vi "8.vi"() -> ()   [LabVIEW 2017]
panel:
  out "毫秒计时值":u32
  in  "开始":bool
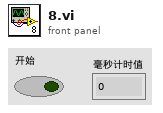
[diagram p1: front panel]
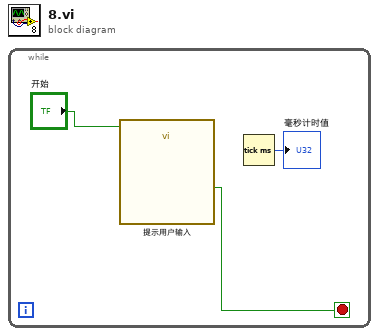
[diagram p0: block diagram]
diagram:
  n1 = while {
    stop <- w2 stop-if-true
    n2 = call "提示用户输入"("Enable"="开始") -> ("确定"=w2:bool)  [unwired: 16 in, 2 out]
    n3 = Tick Count (ms)() -> (millisecond timer value=→"毫秒计时值":u32)
  }
